vi "Begin.vi"(8 "error in":errorcluster) -> (0 "error out":errorcluster)   [LabVIEW 2020]
doc: "Called before other user functions, this VI is expected to open initial I/O refnums, load in file data, and do all program initialization. Notice that the <B>error out</B> terminal is simply used for data flow. Wiring it to other structures or subVIs ensures that this VI runs first."
uses:
  <vilib>/Rock Robotics/WPI/DriverStation/WPI_DriverStationRobotMode2.ctl
  <vilib>/Rock Robotics/WPI/Joystick/WPI_JoystickDeviceEnum.ctl
  <vilib>/Rock Robotics/SystemInterfaces/i2clib/i2c_bus.ctl
  <vilib>/Rock Robotics/WPI/Solenoid/WPI_SolenoidChannel.ctl
  <vilib>/Rock Robotics/SystemInterfaces/DIO/FPGA_DIOChannel.ctl
  Robot Global Data.vi
  <vilib>/Rock Robotics/Network Tables/NT Write String Array.vi
  <vilib>/Rock Robotics/WPI/ThirdParty/Phoenix-LabVIEW/Motor Controller/Get/CTRE_Phoenix_MotorController_GetSelectedSensorData.vi
  <vilib>/Rock Robotics/WPI/Solenoid/WPI_SolenoidOpenDouble.vi
  <vilib>/Rock Robotics/WPI/Switch/WPI_SwitchOpenLimit.vi
  <vilib>/Rock Robotics/WPI/Switch/WPI_SwitchOpenCounting.vi
  <vilib>/Rock Robotics/WPI/ThirdParty/Phoenix-LabVIEW/Motor Controller/Get/CTRE_Phoenix_MotorController_IntegratedSensorData_TalonFX.vi
  GlobalAutonVariables.vi
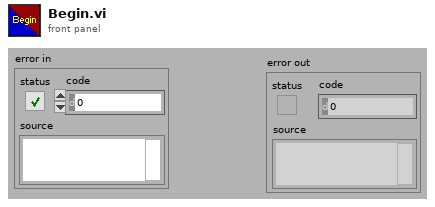
[diagram p1: front panel]
types:
  T1 = enum16{"open", "replace", "create", "open or create", "replace or create", "replace or create with confirmation"}
  T2 = typedef "FPGA_DIOChannel.ctl" = enum8{"DIO 0", "DIO 1", "DIO 2", "DIO 3", "DIO 4", "DIO 5", "DIO 6", "DIO 7", "DIO 8", "DIO 9", "DIO MXP 0", "DIO MXP 1", "DIO MXP 2", "DIO MXP 3", "DIO MXP 4", "DIO MXP 5", "DIO MXP 6", "DIO MXP 7", "DIO MXP 8", "DIO MXP 9", "DIO MXP 10", "DIO MXP 11", "DIO MXP 12", "DIO MXP 13", "DIO MXP 14", "DIO MXP 15", "SPI Port CS1", "SPI Port CS2", "SPI Port CS3", "SPI Port MISO", "SPI Port MOSI", "Invalid"}
  T3 = typedef "WPI_SolenoidChannel.ctl" = enum8{"Solenoid 0", "Solenoid 1", "Solenoid 2", "Solenoid 3", "Solenoid 4", "Solenoid 5", "Solenoid 6", "Solenoid 7", "Solenoid 8", "Solenoid 9", "Solenoid 10", "Solenoid 11", "Solenoid 12", "Solenoid 13", "Solenoid 14", "Solenoid 15", "Invalid"}
  T4 = typedef "i2c_bus.ctl" = enum16{"I2C On-Board", "I2C MXP", "Invalid"}
  T5 = typedef "WPI_JoystickDeviceEnum.ctl" = enum16{"USB 0", "USB 1", "USB 2", "USB 3", "USB 4", "USB 5"}
  T6 = typedef "WPI_DriverStationRobotMode2.ctl" = enum16{"Autonomous Disabled", "Autonomous Enabled", "Teleop Disabled", "Teleop Enabled", "Disconnected", "Finish", "Test Disabled", "Test Enabled", "Emergency Stopped"}
  T7 = typedef "WPI_CompressorDevRef.ctl" = cluster{"DevStatus":errorcluster, "Pneumatics Control Module":u8}
  T8 = typedef "WPI_SolenoidDevRef.ctl" = cluster{"DevStatus":errorcluster, "Pneumatics Control Module":u8, "Forward Solenoid Channel":T3, "Reverse Solenoid Channel":T3}
  T9 = typedef "WPI_JoystickDevRef.ctl" = cluster{"Device":T5}
  T10 = typedef "WPI_MotorControlDeviceRef.ctl" = cluster{"DeviceStatus":errorcluster, "Type":T11, "PWM":cluster{"PWM Channel":T12, "DeadBand":T13}, "CAN":cluster{"Device Number":u8, "SetOutput VI Ref":variant, "GetOutput VI Ref":variant, "Enable VI Ref":variant, "Disable VI Ref":variant, "Data":variant}, "Invert":bool, "DIO PWM":cluster{"PWM \"Enable\" Channel":T12, "DIOChannel":T2, "PWM Rate":dbl}}
  T11 = typedef "WPI_MotorControlType.ctl" = enum16{"PWM", "CAN", "DIO PWM"}
  T12 = typedef "FPGA_DIOPWMChannel.ctl" = enum8{"PWM 0", "PWM 1", "PWM 2", "PWM 3", "PWM 4", "PWM 5", "PWM 6", "PWM 7", "PWM 8", "PWM 9", "PWM MXP 0", "PWM MXP 1", "PWM MXP 2", "PWM MXP 3", "PWM MXP 4", "PWM MXP 5", "PWM MXP 6", "PWM MXP 7", "PWM MXP 8", "PWM MXP 9", "Invalid"}
  T13 = typedef "WPI_PWMDeadband.ctl" = cluster{"Name":string, "maxPositivePwm":i32, "minPositivePwm":i32, "centerPwm":i32, "maxNegativePwm":i32, "minNegativePwm":i32, "angularRange":u16}
  T14 = typedef "Color Sensor V3 DevRef.ctl" = cluster{"I2CDevRef":T15}
  T15 = typedef "WPI_I2CDevRef.ctl" = cluster{"DevStatus":errorcluster, "Device Address":u8, "Handle":i32, "I2C Bus":T4}
  T16 = typedef "CTRE_PigeonIMU_DeviceRef.ctl" = cluster{"DeviceStatus":errorcluster, "Device Number":u8, "Type":T17, "Device ID":u32, "Handle":u64, "UsageFrame":u32, "Library Path":path}
  T17 = typedef "CTRE_PigeonIMU_ConnectionType.ctl" = u32
  T18 = typedef "CTRE_Phoenix_CANcoder_DeviceRef.ctl" = cluster{"DeviceStatus":errorcluster, "Device Number":u8, "Handle":u64, "UsageFrame":u32, "Library Path":path}
  T19 = typedef "WPI_SwitchDevRef.ctl" = cluster{"DevStatus":errorcluster, "DIO Channel":T2, "CntIndex":T20, "Normally Closed":bool}
  T20 = typedef "FPGA_CounterCtrSystemIndex.ctl" = enum8{"Ctr 0", "Ctr 1", "Ctr 2", "Ctr 3", "Ctr 4", "Ctr 5", "Ctr 6", "Ctr 7", "Invalid"}
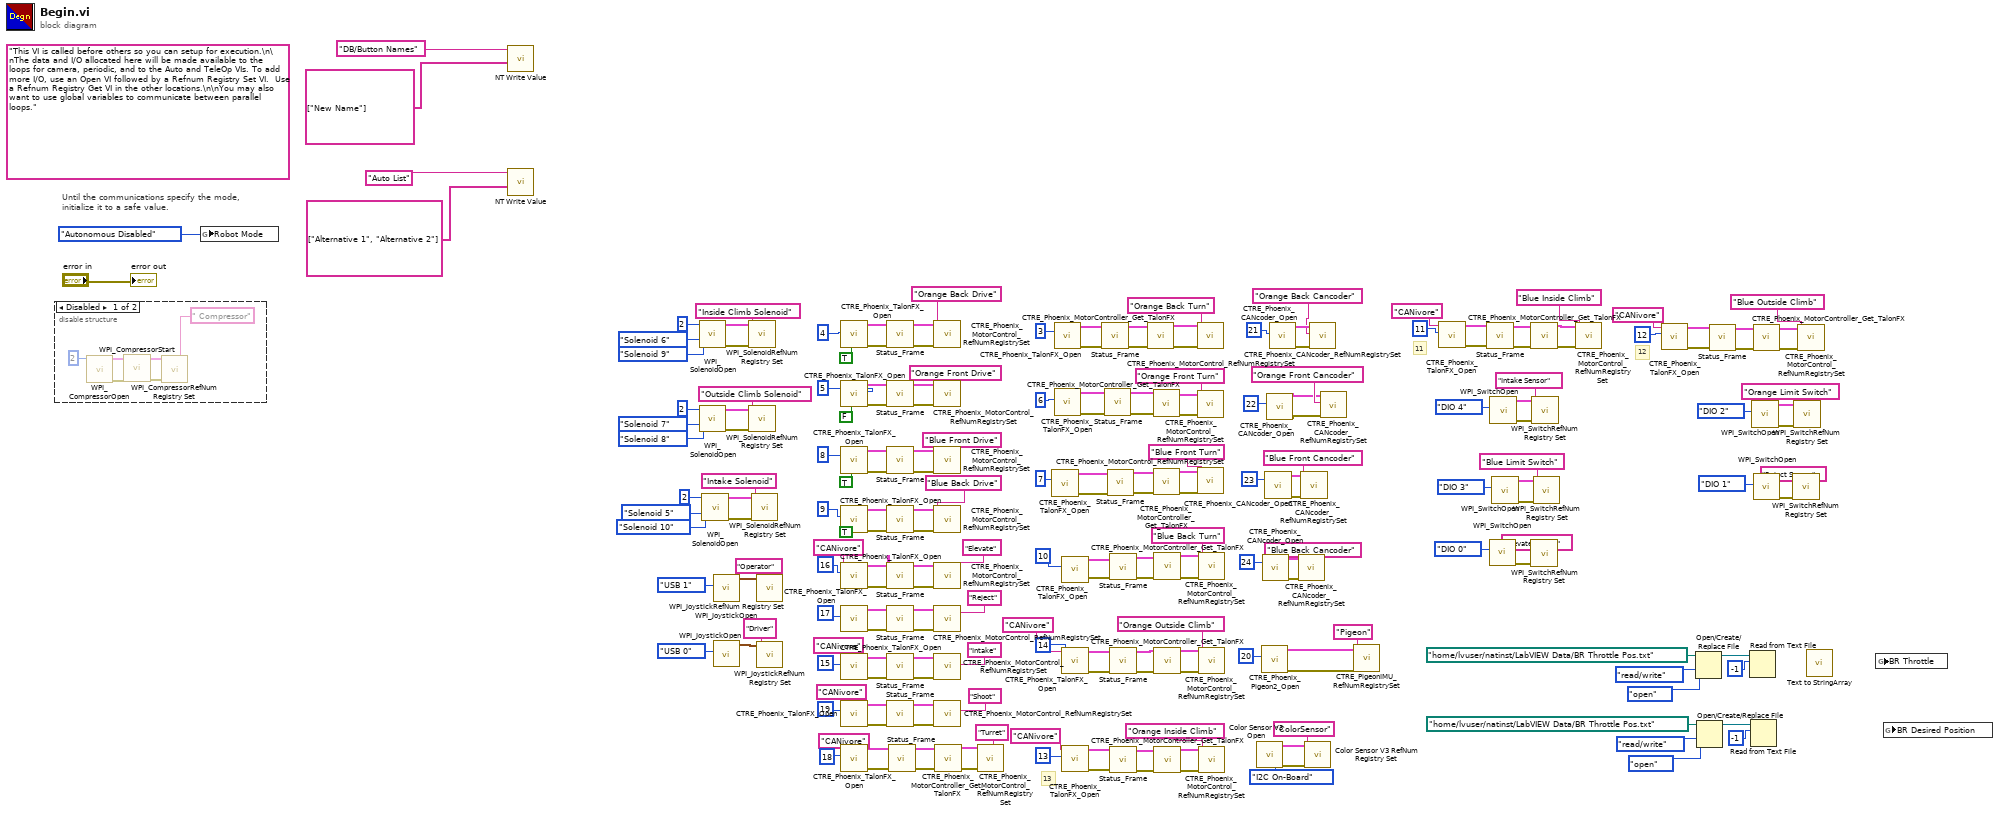
[diagram p0: block diagram]
diagram:
  (unwired) "This VI is called before others so you can setup for execution.\n\nThe data and I/O allocated here will be made available to the loops for camera, periodic, and to the Auto and TeleOp VIs. To add more I/O, use an Open VI followed by a Refnum Registry Set VI.  Use a Refnum Registry Get VI in the other locations.\n\nYou may also want to use global variables to communicate between parallel loops."
  # "13"
  # "12"
  # "11"
  # "Until the communications specify the mode,\ninitialize it to a safe value."
  n1 = disable-structure shown="Disabled" {
    frame Disabled {
      n2 = call <vilib>:"WPI_CompressorOpen.vi"("Pneumatics device (def)"=u8 2) -> ("CompressorDevRef"=w221:T7, "error out"=w222:errorcluster)  [unwired: 13 in]
      n3 = call <vilib>:"WPI_CompressorStart.vi"("error in (no error)"=w222, "CompressorDevRef"=w221) -> ("error out"=w220:errorcluster, "CompressorDevRef"=w219:T7)  [unwired: 8 in]
      n4 = call <vilib>:"WPI_CompressorRefNum Registry Set.vi"("error in (no error)"=w220, "refnum name"=" Compressor", "CompressorDevRef"=w219) -> ()  [unwired: 7 in, 2 out]
    }
    frame Enabled {
    }
  }
  n5 = global write "Robot Global Data.vi" "Robot Mode"(WPI_DriverStationRobotMode2."Autonomous Disabled" ("Robot Mode")) -> ()
  n6 = call-poly <vilib>:"NT Write Value.vi"("String Array"=string[] ["New Name"], "Name"="DB/Button Names") -> ()  [unwired: 9 in, 1 out]
  n7 = call-poly <vilib>:"NT Write Value.vi"("String Array"=string[] ["Alternative 1", "Alternative 2"], "Name"="Auto List") -> ()  [unwired: 9 in, 1 out]
  n8 = call-poly <vilib>:"WPI_SolenoidOpen.vi"("Reverse Solenoid Channel"=WPI_SolenoidChannel."Solenoid 9", "Forward Solenoid Channel"=WPI_SolenoidChannel."Solenoid 6", "Pneumatics Device (def)"=u8 2) -> ("error out"=w165:errorcluster, "SolenoidDevRef"=w164:T8)  [unwired: 7 in]
  n9 = call-poly <vilib>:"WPI_SolenoidOpen.vi"("Reverse Solenoid Channel"=WPI_SolenoidChannel."Solenoid 8", "Forward Solenoid Channel"=WPI_SolenoidChannel."Solenoid 7", "Pneumatics Device (def)"=u8 2) -> ("error out"=w162:errorcluster, "SolenoidDevRef"=w161:T8)  [unwired: 7 in]
  n10 = call-poly <vilib>:"WPI_SolenoidOpen.vi"("Reverse Solenoid Channel"=WPI_SolenoidChannel."Solenoid 10", "Forward Solenoid Channel"=WPI_SolenoidChannel."Solenoid 5", "Pneumatics Device (def)"=u8 2) -> ("error out"=w159:errorcluster, "SolenoidDevRef"=w158:T8)  [unwired: 7 in]
  n11 = call <vilib>:"WPI_JoystickOpen.vi"("JoystickDevice"=WPI_JoystickDeviceEnum."USB 1") -> ("JoystickDevRef"=w206:T9)  [unwired: 10 in]
  n12 = call <vilib>:"WPI_JoystickOpen.vi"("JoystickDevice"=WPI_JoystickDeviceEnum."USB 0") -> ("JoystickDevRef"=w214:T9)  [unwired: 10 in]
  n13 = call <vilib>:"WPI_SolenoidRefNum Registry Set.vi"("error in (no error)"=w165, "refnum name"="Inside Climb Solenoid", "SolenoidDevRef"=w164) -> ()  [unwired: 7 in, 2 out]
  n14 = call <vilib>:"WPI_SolenoidRefNum Registry Set.vi"("error in (no error)"=w162, "refnum name"="Outside Climb Solenoid", "SolenoidDevRef"=w161) -> ()  [unwired: 7 in, 2 out]
  n15 = call <vilib>:"WPI_SolenoidRefNum Registry Set.vi"("error in (no error)"=w159, "refnum name"="Intake Solenoid", "SolenoidDevRef"=w158) -> ()  [unwired: 7 in, 2 out]
  n16 = call <vilib>:"WPI_JoystickRefNum Registry Set.vi"("refnum name"="Operator", "JoystickDevRef"=w206) -> ()  [unwired: 8 in, 2 out]
  n17 = call <vilib>:"WPI_JoystickRefNum Registry Set.vi"("refnum name"="Driver", "JoystickDevRef"=w214) -> ()  [unwired: 8 in, 2 out]
  n18 = call <vilib>:"CTRE_Phoenix_TalonFX_Open.vi"("Invert"=TRUE, "Device Number"=u8 4) -> ("error out"=w85:errorcluster, "PhoenixMotorControlDevRef"=w86:T10)  [unwired: 8 in]
  n19 = call <vilib>:"CTRE_Phoenix_TalonFX_Open.vi"("Invert"=FALSE, "Device Number"=u8 5) -> ("error out"=w78:errorcluster, "PhoenixMotorControlDevRef"=w77:T10)  [unwired: 8 in]
  n20 = call <vilib>:"CTRE_Phoenix_TalonFX_Open.vi"("Invert"=TRUE, "Device Number"=u8 8) -> ("error out"=w82:errorcluster, "PhoenixMotorControlDevRef"=w79:T10)  [unwired: 8 in]
  n21 = call <vilib>:"CTRE_Phoenix_TalonFX_Open.vi"("Invert"=TRUE, "Device Number"=u8 9) -> ("error out"=w71:errorcluster, "PhoenixMotorControlDevRef"=w74:T10)  [unwired: 8 in]
  n22 = call <vilib>:"CTRE_Phoenix_TalonFX_Open.vi"("Device Number"=u8 16, "CAN Bus"="CANivore") -> ("error out"=w67:errorcluster, "PhoenixMotorControlDevRef"=w70:T10)  [unwired: 8 in]
  n23 = call <vilib>:"CTRE_Phoenix_TalonFX_Open.vi"("Device Number"=u8 17) -> ("error out"=w63:errorcluster, "PhoenixMotorControlDevRef"=w66:T10)  [unwired: 9 in]
  n24 = call <vilib>:"CTRE_Phoenix_TalonFX_Open.vi"("Device Number"=u8 15, "CAN Bus"="CANivore") -> ("error out"=w59:errorcluster, "PhoenixMotorControlDevRef"=w62:T10)  [unwired: 8 in]
  n25 = call <vilib>:"CTRE_Phoenix_TalonFX_Open.vi"("Device Number"=u8 19, "CAN Bus"="CANivore") -> ("error out"=w55:errorcluster, "PhoenixMotorControlDevRef"=w58:T10)  [unwired: 8 in]
  n26 = call <vilib>:"CTRE_Phoenix_TalonFX_Open.vi"("Device Number"=u8 18, "CAN Bus"="CANivore") -> ("error out"=w52:errorcluster, "PhoenixMotorControlDevRef"=w53:T10)  [unwired: 8 in]
  n27 = call "Status_Frame.vi"("error in (no error)"=w85, "Motor Control DevRef"=w86) -> ("error out"=w84:errorcluster, "PhoenixMotorControlDevRef"=w83:T10)  [unwired: 8 in]
  n28 = call "Status_Frame.vi"("error in (no error)"=w78, "Motor Control DevRef"=w77) -> ("error out"=w75:errorcluster, "PhoenixMotorControlDevRef"=w76:T10)  [unwired: 8 in]
  n29 = call "Status_Frame.vi"("error in (no error)"=w82, "Motor Control DevRef"=w79) -> ("error out"=w81:errorcluster, "PhoenixMotorControlDevRef"=w80:T10)  [unwired: 8 in]
  n30 = call "Status_Frame.vi"("error in (no error)"=w71, "Motor Control DevRef"=w74) -> ("error out"=w72:errorcluster, "PhoenixMotorControlDevRef"=w73:T10)  [unwired: 8 in]
  n31 = call "Status_Frame.vi"("error in (no error)"=w67, "Motor Control DevRef"=w70) -> ("error out"=w68:errorcluster, "PhoenixMotorControlDevRef"=w69:T10)  [unwired: 8 in]
  n32 = call "Status_Frame.vi"("error in (no error)"=w63, "Motor Control DevRef"=w66) -> ("error out"=w64:errorcluster, "PhoenixMotorControlDevRef"=w65:T10)  [unwired: 8 in]
  n33 = call "Status_Frame.vi"("error in (no error)"=w59, "Motor Control DevRef"=w62) -> ("error out"=w60:errorcluster, "PhoenixMotorControlDevRef"=w61:T10)  [unwired: 8 in]
  n34 = call "Status_Frame.vi"("error in (no error)"=w55, "Motor Control DevRef"=w58) -> ("error out"=w56:errorcluster, "PhoenixMotorControlDevRef"=w57:T10)  [unwired: 8 in]
  n35 = call "Status_Frame.vi"("error in (no error)"=w52, "Motor Control DevRef"=w53) -> ("error out"=w13:errorcluster, "PhoenixMotorControlDevRef"=w14:T10)  [unwired: 8 in]
  n36 = call <vilib>:"CTRE_Phoenix_MotorControl_RefNumRegistrySet.vi"("error in (no error)"=w84, "refnum name"="Orange Back Drive", "PhoenixMotorControlDevRef"=w83) -> ()  [unwired: 7 in, 2 out]
  n37 = call <vilib>:"CTRE_Phoenix_MotorControl_RefNumRegistrySet.vi"("error in (no error)"=w75, "refnum name"="Orange Front Drive", "PhoenixMotorControlDevRef"=w76) -> ()  [unwired: 7 in, 2 out]
  n38 = call <vilib>:"CTRE_Phoenix_MotorControl_RefNumRegistrySet.vi"("error in (no error)"=w81, "refnum name"="Blue Front Drive", "PhoenixMotorControlDevRef"=w80) -> ()  [unwired: 7 in, 2 out]
  n39 = call <vilib>:"CTRE_Phoenix_MotorControl_RefNumRegistrySet.vi"("error in (no error)"=w72, "refnum name"="Blue Back Drive", "PhoenixMotorControlDevRef"=w73) -> ()  [unwired: 7 in, 2 out]
  n40 = call <vilib>:"CTRE_Phoenix_MotorControl_RefNumRegistrySet.vi"("error in (no error)"=w68, "refnum name"="Elevate", "PhoenixMotorControlDevRef"=w69) -> ()  [unwired: 7 in, 2 out]
  n41 = call <vilib>:"CTRE_Phoenix_MotorControl_RefNumRegistrySet.vi"("error in (no error)"=w64, "refnum name"="Reject", "PhoenixMotorControlDevRef"=w65) -> ()  [unwired: 7 in, 2 out]
  n42 = call <vilib>:"CTRE_Phoenix_MotorControl_RefNumRegistrySet.vi"("error in (no error)"=w60, "refnum name"="Intake", "PhoenixMotorControlDevRef"=w61) -> ()  [unwired: 7 in, 2 out]
  n43 = call <vilib>:"CTRE_Phoenix_MotorControl_RefNumRegistrySet.vi"("error in (no error)"=w56, "refnum name"="Shoot", "PhoenixMotorControlDevRef"=w57) -> ()  [unwired: 7 in, 2 out]
  n44 = call-poly <vilib>:"CTRE_Phoenix_MotorController_Get_TalonFX.vi"("PhoenixMotorControlDevRef"=w14, "error in"=w13) -> ("PhoenixMotorControlDevRef"=w11:T10, "error out"=w12:errorcluster)  [unwired: 9 in, 3 out]
  n45 = call <vilib>:"CTRE_Phoenix_MotorControl_RefNumRegistrySet.vi"("error in (no error)"=w12, "refnum name"="Turret", "PhoenixMotorControlDevRef"=w11) -> ()  [unwired: 7 in, 2 out]
  n46 = call <vilib>:"CTRE_Phoenix_TalonFX_Open.vi"("Device Number"=u8 7) -> ("error out"=w40:errorcluster, "PhoenixMotorControlDevRef"=w43:T10)  [unwired: 9 in]
  n47 = call <vilib>:"CTRE_Phoenix_TalonFX_Open.vi"("Device Number"=u8 3) -> ("error out"=w48:errorcluster, "PhoenixMotorControlDevRef"=w51:T10)  [unwired: 9 in]
  n48 = call <vilib>:"CTRE_Phoenix_TalonFX_Open.vi"("Device Number"=u8 6) -> ("error out"=w44:errorcluster, "PhoenixMotorControlDevRef"=w47:T10)  [unwired: 9 in]
  n49 = call <vilib>:"CTRE_Phoenix_TalonFX_Open.vi"("Device Number"=u8 10) -> ("error out"=w36:errorcluster, "PhoenixMotorControlDevRef"=w37:T10)  [unwired: 9 in]
  n50 = call <vilib>:"CTRE_Phoenix_TalonFX_Open.vi"("Device Number"=u8 14, "CAN Bus"="CANivore") -> ("error out"=w26:errorcluster, "PhoenixMotorControlDevRef"=w27:T10)  [unwired: 8 in]
  n51 = call <vilib>:"CTRE_Phoenix_TalonFX_Open.vi"("Device Number"=u8 13, "CAN Bus"="CANivore") -> ("error out"=w24:errorcluster, "PhoenixMotorControlDevRef"=w25:T10)  [unwired: 8 in]
  n52 = call "Status_Frame.vi"("error in (no error)"=w48, "Motor Control DevRef"=w51) -> ("error out"=w49:errorcluster, "PhoenixMotorControlDevRef"=w50:T10)  [unwired: 8 in]
  n53 = call "Status_Frame.vi"("error in (no error)"=w44, "Motor Control DevRef"=w47) -> ("error out"=w45:errorcluster, "PhoenixMotorControlDevRef"=w46:T10)  [unwired: 8 in]
  n54 = call "Status_Frame.vi"("error in (no error)"=w40, "Motor Control DevRef"=w43) -> ("error out"=w41:errorcluster, "PhoenixMotorControlDevRef"=w42:T10)  [unwired: 8 in]
  n55 = call "Status_Frame.vi"("error in (no error)"=w36, "Motor Control DevRef"=w37) -> ("error out"=w38:errorcluster, "PhoenixMotorControlDevRef"=w39:T10)  [unwired: 8 in]
  n56 = call "Status_Frame.vi"("error in (no error)"=w26, "Motor Control DevRef"=w27) -> ("error out"=w34:errorcluster, "PhoenixMotorControlDevRef"=w35:T10)  [unwired: 8 in]
  n57 = call "Status_Frame.vi"("error in (no error)"=w24, "Motor Control DevRef"=w25) -> ("error out"=w32:errorcluster, "PhoenixMotorControlDevRef"=w33:T10)  [unwired: 8 in]
  n58 = call-poly <vilib>:"CTRE_Phoenix_MotorController_Get_TalonFX.vi"("PhoenixMotorControlDevRef"=w50, "error in"=w49) -> ("PhoenixMotorControlDevRef"=w102:T10, "error out"=w204:errorcluster)  [unwired: 10 in, 2 out]
  n59 = call-poly <vilib>:"CTRE_Phoenix_MotorController_Get_TalonFX.vi"("PhoenixMotorControlDevRef"=w46, "error in"=w45) -> ("PhoenixMotorControlDevRef"=w197:T10, "error out"=w198:errorcluster)  [unwired: 10 in, 2 out]
  n60 = call-poly <vilib>:"CTRE_Phoenix_MotorController_Get_TalonFX.vi"("PhoenixMotorControlDevRef"=w42, "error in"=w41) -> ("PhoenixMotorControlDevRef"=w108:T10, "error out"=w103:errorcluster)  [unwired: 10 in, 2 out]
  n61 = call-poly <vilib>:"CTRE_Phoenix_MotorController_Get_TalonFX.vi"("PhoenixMotorControlDevRef"=w39, "error in"=w38) -> ("PhoenixMotorControlDevRef"=w104:T10, "error out"=w185:errorcluster)  [unwired: 10 in, 2 out]
  n62 = call-poly <vilib>:"CTRE_Phoenix_MotorController_Get_TalonFX.vi"("PhoenixMotorControlDevRef"=w35, "error in"=w34) -> ("PhoenixMotorControlDevRef"=w105:T10, "error out"=w122:errorcluster)  [unwired: 10 in, 2 out]
  n63 = call-poly <vilib>:"CTRE_Phoenix_MotorController_Get_TalonFX.vi"("PhoenixMotorControlDevRef"=w33, "error in"=w32) -> ("PhoenixMotorControlDevRef"=w107:T10, "error out"=w119:errorcluster)  [unwired: 10 in, 2 out]
  n64 = call <vilib>:"CTRE_Phoenix_MotorControl_RefNumRegistrySet.vi"("error in (no error)"=w204, "refnum name"="Orange Back Turn", "PhoenixMotorControlDevRef"=w102) -> ()  [unwired: 7 in, 2 out]
  n65 = call <vilib>:"CTRE_Phoenix_MotorControl_RefNumRegistrySet.vi"("error in (no error)"=w198, "refnum name"="Orange Front Turn", "PhoenixMotorControlDevRef"=w197) -> ()  [unwired: 7 in, 2 out]
  n66 = call <vilib>:"CTRE_Phoenix_MotorControl_RefNumRegistrySet.vi"("error in (no error)"=w103, "refnum name"="Blue Front Turn", "PhoenixMotorControlDevRef"=w108) -> ()  [unwired: 7 in, 2 out]
  n67 = call <vilib>:"CTRE_Phoenix_MotorControl_RefNumRegistrySet.vi"("error in (no error)"=w185, "refnum name"="Blue Back Turn", "PhoenixMotorControlDevRef"=w104) -> ()  [unwired: 7 in, 2 out]
  n68 = call <vilib>:"CTRE_Phoenix_MotorControl_RefNumRegistrySet.vi"("error in (no error)"=w122, "refnum name"="Orange Outside Climb", "PhoenixMotorControlDevRef"=w105) -> ()  [unwired: 7 in, 2 out]
  n69 = call <vilib>:"CTRE_Phoenix_MotorControl_RefNumRegistrySet.vi"("error in (no error)"=w119, "refnum name"="Orange Inside Climb", "PhoenixMotorControlDevRef"=w107) -> ()  [unwired: 7 in, 2 out]
  n70 = call <vilib>:"Color Sensor V3 Open.vi"("I2C Bus"=i2c_bus."I2C On-Board") -> ("error out"=w169:errorcluster, "ColorSensorDevRef"=w168:T14)  [unwired: 9 in]
  n71 = call <vilib>:"CTRE_Phoenix_Pigeon2_Open.vi"("Device Number"=u8 20) -> ("error out"=w15:errorcluster, "PigeonIMUDevRef"=w16:T16)  [unwired: 9 in]
  n72 = call <vilib>:"CTRE_Phoenix_CANcoder_Open.vi"("Device Number"=u8 24) -> ("error out"=w97:errorcluster, "CTRE_CANcoder_DeviceRef"=w98:T18)  [unwired: 9 in]
  n73 = call <vilib>:"CTRE_Phoenix_CANcoder_Open.vi"("Device Number"=u8 23) -> ("error out"=w99:errorcluster, "CTRE_CANcoder_DeviceRef"=w100:T18)  [unwired: 9 in]
  n74 = call <vilib>:"CTRE_Phoenix_CANcoder_Open.vi"("Device Number"=u8 22) -> ("error out"=w96:errorcluster, "CTRE_CANcoder_DeviceRef"=w95:T18)  [unwired: 9 in]
  n75 = call <vilib>:"CTRE_Phoenix_CANcoder_Open.vi"("Device Number"=u8 21) -> ("error out"=w18:errorcluster, "CTRE_CANcoder_DeviceRef"=w19:T18)  [unwired: 9 in]
  n76 = call <vilib>:"CTRE_Phoenix_CANcoder_RefNumRegistrySet.vi"("error in (no error)"=w97, "refnum name"="Blue Back Cancoder", "CTRE_CANcoder_DeviceRef"=w98) -> ()  [unwired: 7 in, 2 out]
  n77 = call <vilib>:"CTRE_Phoenix_CANcoder_RefNumRegistrySet.vi"("error in (no error)"=w99, "refnum name"="Blue Front Cancoder", "CTRE_CANcoder_DeviceRef"=w100) -> ()  [unwired: 7 in, 2 out]
  n78 = call <vilib>:"Color Sensor V3 RefNum Registry Set.vi"("error in (no error)"=w169, "refnum name"="ColorSensor", "ColorSensorDevRef"=w168) -> ()  [unwired: 7 in, 2 out]
  n79 = call <vilib>:"CTRE_Phoenix_CANcoder_RefNumRegistrySet.vi"("error in (no error)"=w18, "refnum name"="Orange Back Cancoder", "CTRE_CANcoder_DeviceRef"=w19) -> ()  [unwired: 7 in, 2 out]
  n80 = call <vilib>:"CTRE_Phoenix_CANcoder_RefNumRegistrySet.vi"("error in (no error)"=w96, "refnum name"="Orange Front Cancoder", "CTRE_CANcoder_DeviceRef"=w95) -> ()  [unwired: 7 in, 2 out]
  n81 = call <vilib>:"CTRE_PigeonIMU_RefNumRegistrySet.vi"("error in (no error)"=w15, "refnum name"="Pigeon", "PigeonIMUDevRef"=w16) -> ()  [unwired: 7 in, 2 out]
  n82 = call <vilib>:"CTRE_Phoenix_TalonFX_Open.vi"("Device Number"=u8 11, "CAN Bus"="CANivore") -> ("error out"=w20:errorcluster, "PhoenixMotorControlDevRef"=w21:T10)  [unwired: 8 in]
  n83 = call "Status_Frame.vi"("error in (no error)"=w20, "Motor Control DevRef"=w21) -> ("error out"=w28:errorcluster, "PhoenixMotorControlDevRef"=w29:T10)  [unwired: 8 in]
  n84 = call-poly <vilib>:"WPI_SwitchOpen.vi"("DIO Channel"=FPGA_DIOChannel."DIO 0") -> ("error out"=w147:errorcluster, "SwitchDevRef"=w146:T19)  [unwired: 9 in]
  n85 = call-poly <vilib>:"WPI_SwitchOpen.vi"("DIO Channel"=FPGA_DIOChannel."DIO 4") -> ("error out"=w126:errorcluster, "SwitchDevRef"=w125:T19)  [unwired: 9 in]
  n86 = call-poly <vilib>:"WPI_SwitchOpen.vi"("DIO Channel"=FPGA_DIOChannel."DIO 3") -> ("error out"=w130:errorcluster, "SwitchDevRef"=w129:T19)  [unwired: 9 in]
  n87 = call-poly <vilib>:"CTRE_Phoenix_MotorController_Get_TalonFX.vi"("PhoenixMotorControlDevRef"=w29, "error in"=w28) -> ("PhoenixMotorControlDevRef"=w111:T10, "error out"=w112:errorcluster)  [unwired: 10 in, 2 out]
  n88 = call <vilib>:"WPI_SwitchRefNum Registry Set.vi"("error in (no error)"=w147, "refnum name"="Elevate Sensor", "SwitchDevRef"=w146) -> ()  [unwired: 7 in, 2 out]
  n89 = call <vilib>:"WPI_SwitchRefNum Registry Set.vi"("error in (no error)"=w126, "refnum name"="Intake Sensor", "SwitchDevRef"=w125) -> ()  [unwired: 7 in, 2 out]
  n90 = call <vilib>:"WPI_SwitchRefNum Registry Set.vi"("error in (no error)"=w130, "refnum name"="Blue Limit Switch", "SwitchDevRef"=w129) -> ()  [unwired: 7 in, 2 out]
  n91 = call <vilib>:"CTRE_Phoenix_MotorControl_RefNumRegistrySet.vi"("error in (no error)"=w112, "refnum name"="Blue Inside Climb", "PhoenixMotorControlDevRef"=w111) -> ()  [unwired: 7 in, 2 out]
  n92 = call <vilib>:"CTRE_Phoenix_TalonFX_Open.vi"("Device Number"=u8 12, "CAN Bus"="CANivore") -> ("error out"=w22:errorcluster, "PhoenixMotorControlDevRef"=w23:T10)  [unwired: 8 in]
  n93 = Open/Create/Replace File(file path (use dialog)=path "/home/lvuser/natinst/LabVIEW Data/BR Throttle Pos.txt", operation (0:open)=T1."open", access (0:read/write)=enum16{"read/write", "read-only", "write-only"}."read/write") -> (refnum out=w7:refnum<file>)  [unwired: 3 in, 2 out]
  n94 = Open/Create/Replace File(file path (use dialog)=path "/home/lvuser/natinst/LabVIEW Data/BR Throttle Pos.txt", operation (0:open)=T1."open", access (0:read/write)=enum16{"read/write", "read-only", "write-only"}."read/write") -> (refnum out=w2:refnum<file>)  [unwired: 3 in, 2 out]
  n95 = call "Status_Frame.vi"("error in (no error)"=w22, "Motor Control DevRef"=w23) -> ("error out"=w30:errorcluster, "PhoenixMotorControlDevRef"=w31:T10)  [unwired: 8 in]
  n96 = Read from Text File(file (use dialog)=w7, count=-1) -> ()  [unwired: 2 in, 4 out]
  n97 = Read from Text File(file (use dialog)=w2, count=-1) -> ()  [unwired: 2 in, 4 out]
  n98 = call-poly <vilib>:"WPI_SwitchOpen.vi"("DIO Channel"=FPGA_DIOChannel."DIO 2") -> ("error out"=w134:errorcluster, "SwitchDevRef"=w133:T19)  [unwired: 9 in]
  n99 = call-poly <vilib>:"CTRE_Phoenix_MotorController_Get_TalonFX.vi"("PhoenixMotorControlDevRef"=w31, "error in"=w30) -> ("PhoenixMotorControlDevRef"=w115:T10, "error out"=w116:errorcluster)  [unwired: 10 in, 2 out]
  n100 = call-poly <vilib>:"WPI_SwitchOpen.vi"("DIO Channel"=FPGA_DIOChannel."DIO 1") -> ("error out"=w143:errorcluster, "SwitchDevRef"=w142:T19)  [unwired: 9 in]
  n101 = call <vilib>:"WPI_SwitchRefNum Registry Set.vi"("error in (no error)"=w143, "refnum name"="Reject Sensor", "SwitchDevRef"=w142) -> ()  [unwired: 7 in, 2 out]
  n102 = call <vilib>:"WPI_SwitchRefNum Registry Set.vi"("error in (no error)"=w134, "refnum name"="Orange Limit Switch", "SwitchDevRef"=w133) -> ()  [unwired: 7 in, 2 out]
  n103 = call <vilib>:"CTRE_Phoenix_MotorControl_RefNumRegistrySet.vi"("error in (no error)"=w116, "refnum name"="Blue Outside Climb", "PhoenixMotorControlDevRef"=w115) -> ()  [unwired: 7 in, 2 out]
  n104 = call "Text to StringArray.vi"() -> ()  [unwired: 1 in]
  n105 = global read "GlobalAutonVariables.vi" "BR Throttle"() -> ()  [unwired: 1 in]
  n106 = global read "GlobalAutonVariables.vi" "BR Desired Position"() -> ()  [unwired: 1 in]
  "error out" <- "error in"
